vi "CheckSee.vi"(4 "User Parameter":T1, 5 "Event Data":cluster{"return value":refnum<k24>}, 6 "Control Ref":refnum<k24>, 7 "Event Common Data":T2) -> (1 "Event Data Out":cluster{"return value":refnum<k24>})   [LabVIEW 2018]
uses:
  D:/NI LabVIEW/PowerControlWithAT2/REMOTE_SEE_CONTROLLER/RemoteSeeAbleService.dll
  RemoteSeeAbleService.dll
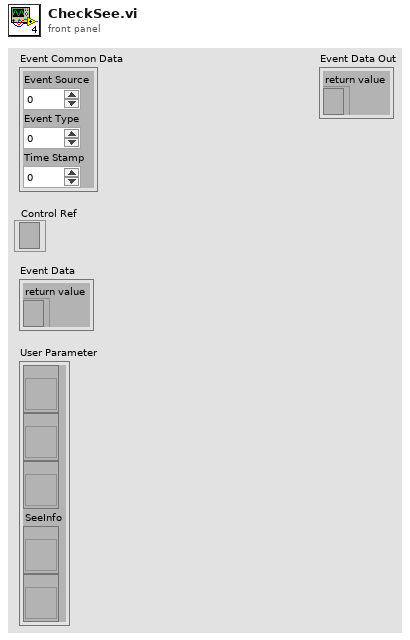
[diagram p1: front panel]
types:
  T1 = cluster{refnum<vi>, refnum<vi>, refnum<vi>, "SeeInfo":refnum<vi>, refnum<vi>}
  T2 = cluster{"Event Source":i32, "Event Type":u32, "Time Stamp":u32}
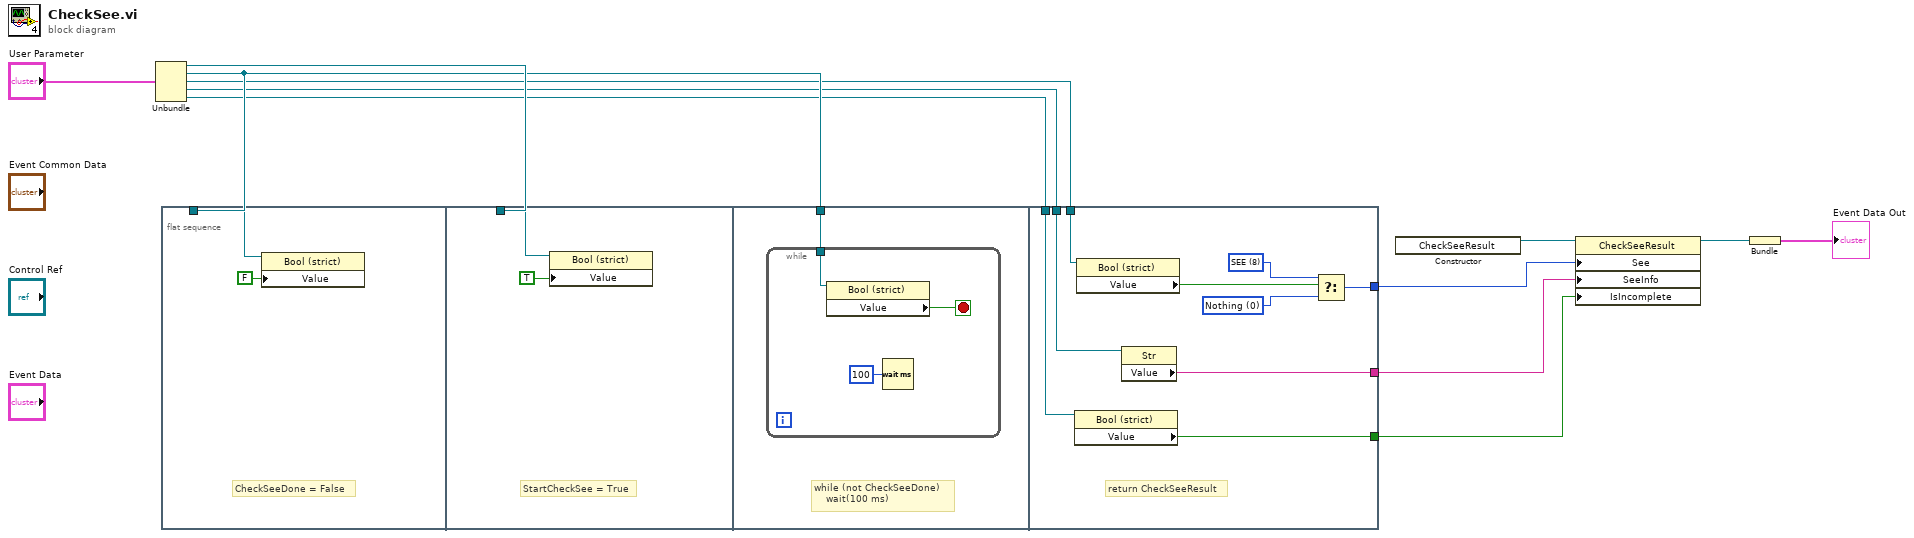
[diagram p0: block diagram]
diagram:
  n1 = Unbundle("User Parameter") -> (w11:refnum<vi>, w10:refnum<vi>, w8:refnum<vi>, "SeeInfo"=w6:refnum<vi>, w4:refnum<vi>)
  n2 = flat-sequence {
    tunnel: w10 -> [w14]
    tunnel: w11 -> [w15]
    tunnel: w10 -> [w17]
    tunnel: w8 -> [w29]
    tunnel: [w25] -> w7
    tunnel: w6 -> [w24]
    tunnel: [w23] -> w5
    tunnel: w4 -> [w22]
    tunnel: [w21] -> w3
    frame #0 {
      # "CheckSeeDone = False"
      n3 = property class="Bool (strict)"(reference=w14, "Value"=FALSE) -> ()  [unwired: 1 in, 2 out]
    }
    frame #1 {
      # "StartCheckSee = True"
      n4 = property class="Bool (strict)"(reference=w15, "Value"=TRUE) -> ()  [unwired: 1 in, 2 out]
    }
    frame #2 {
      # "while (not CheckSeeDone)\n    wait(100 ms)"
      n5 = while {
        tunnel: w17 -> [w19]
        stop <- w20 stop-if-true
        n6 = property class="Bool (strict)"(reference=w19) -> ("Value"=w20:bool)  [unwired: 1 in, 2 out]
        n7 = Wait (ms)(milliseconds to wait=u32 100) -> ()  [unwired: 1 out]
      }
    }
    frame #3 {
      w27 = 8 items=["Nothing", "SEL", "SEU", "SEFI", "CatastrophicUpset", "SET", "SEB", "SEGR", "SEE"] ("See")
      w26 = 0 items=["Nothing", "SEL", "SEU", "SEFI", "CatastrophicUpset", "SET", "SEB", "SEGR", "SEE"] ("See")
      # "return CheckSeeResult"
      n8 = property class="Bool (strict)"(reference=w22) -> ("Value"=w21:bool)  [unwired: 1 in, 2 out]
      n9 = property class="Bool (strict)"(reference=w29) -> ("Value"=w28:bool)  [unwired: 1 in, 2 out]
      n10 = property class="Str"(reference=w24) -> ("Value"=w23:string)  [unwired: 1 in, 2 out]
      n11 = Select(t=w27, s=w28, f=w26) -> (s? t:f=w25:i32)
    }
  }
  n12 = constructor class="CheckSeeResult"() -> (reference out=w9:refnum<k24>)  [unwired: 3 in, 2 out]
  n13 = property class="CheckSeeResult"(reference=w9, "See"=w7, "SeeInfo"=w5, "IsIncomplete"=w3) -> (reference out=w2:refnum<k24>)  [unwired: 1 in, 1 out]
  n14 = Bundle("new reference"=w2) -> (→"Event Data Out":cluster{"new reference":refnum<k24>})  [unwired: 1 in]
